vi "LinxServoGetChans.vi"(8 "Error In":errorcluster, 11 "LINX Resource":T1) -> (0 "Error Out":errorcluster, 1 "Num Servo Chans":i32, 2 "Servo Channels":u8[](array[numeric]), 3 "LINX Resource":T1)   [LabVIEW 2020, in "LMH-LINX.lvlib" / "Local IO.lvlib"]
uses:
  Local IO.lvlib
  Type Defs/LINX Ref.ctl
  Type Defs/Platform.ctl
  Device/Type Defs/LINX Device Config.ctl
  Type Defs/Interface.ctl
  Device/Type Defs/TCP Config.ctl
  Device/Type Defs/Channels.ctl
  Type Defs/Error Type.ctl
  LMH-LINX.lvlib
  <vilib>/MakerHub/LINX/Resources/liblinxdevice.dll
  Device/Device.lvlib
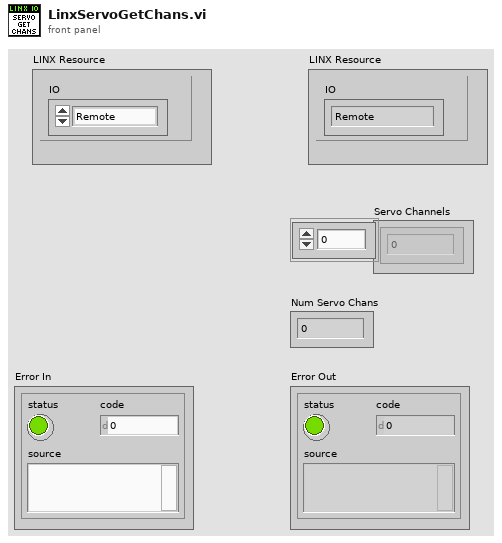
[diagram p1: front panel]
types:
  T1 = typedef "LMH-LINX.lvlib/LINX Ref.ctl" = cluster{"IO":T2, "LINX Device Config":T3}
  T2 = typedef "LMH-LINX.lvlib/Platform.ctl" = enum16{"Remote", "Local"}
  T3 = typedef "Device.lvlib/LINX Device Config.ctl" = cluster{"Interface":T4, "COM Port":refnum<visa-resource-name>, "TCP Configuration":T5, "Device Family":u8, "Device ID":u8, "Device Name":string, "TCP Ref":refnum<k5>, "Channels":T6}
  T4 = typedef "LMH-LINX.lvlib/Interface.ctl" = enum16{"Serial", "TCP"}
  T5 = typedef "Device.lvlib/TCP Config.ctl" = cluster{"IP Address":string, "Port":u16}
  T6 = typedef "LMH-LINX.lvlib/Channels.ctl" = cluster{"DI":u8[], "DO":u8[], "AI":u8[], "AO":u8[], "PWM":u8[], "QE":u8[], "UART":u8[], "I2C 2":u8[], "SPI":u8[], "CAN":u8[], "Servo":u8[], "AI Ref (V)":dbl, "AI Resolution (Bits)":u8, "AO Ref (V)":dbl, "AO Resolution (Bits)":u8}
  T7 = typedef "LMH-LINX.lvlib/Error Type.ctl" = enum16{"Unknown", "Timeout", "Corrupt Return Packet", "Unable To Connect", "Command Not Supported", "Channel DNE", "Invalid COM Config", "Firmware Version Mismatch", "myRIO Support", "CMD Specific Error", "Local IO Not Supported"}
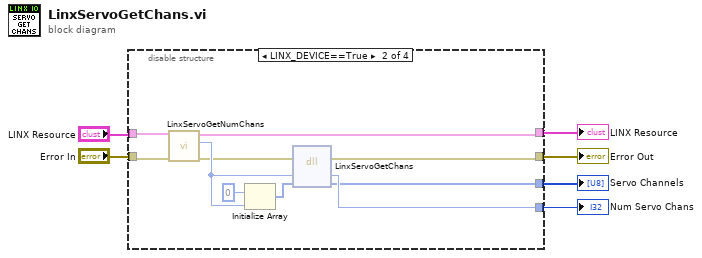
[diagram p0: block diagram]
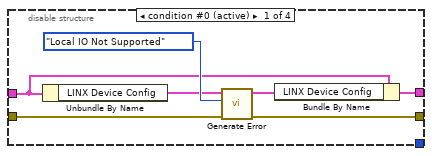
[diagram p2: hidden frame]
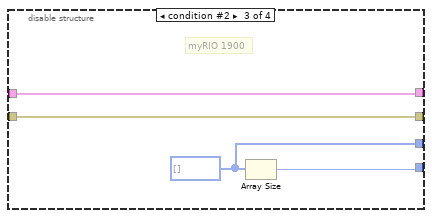
[diagram p3: hidden frame]
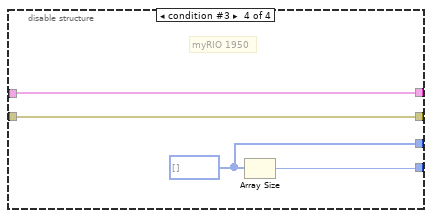
[diagram p4: hidden frame]
diagram:
  n1 = disable-structure shown="LINX_DEVICE==True" {
    disable-tunnel: [w7 w16 w26 w28] -> w3
    disable-tunnel: "LINX Resource" -> [w9 w19 w26 w28]
    disable-tunnel: "Error In" -> [w12 w18 w27 w31]
    disable-tunnel: [w11 w17 w27 w31] -> w5
    disable-tunnel: [_ w15 w25 w30] -> w2
    disable-tunnel: [_ w14 w24 w29] -> w1
    frame condition #0 (active) {
      n2 = Unbundle By Name(w9) -> ("LINX Device Config"=w10:T3)
      n3 = call "Generate Error.vi"("Error In"=w12, "Error Type"=Error_Type."Local IO Not Supported", "LINX Device Config"=w10) -> ("Error Out"=w11:errorcluster, "Dup LINX Device Config"=w8:T3)  [unwired: 7 in]
      n4 = Bundle By Name(cluster=w9, "LINX Device Config"=w8) -> (w7:T1)
    }
    frame condition #1 {
      n5 = call "LinxServoGetNumChans.vi"("Error In"=w18, "LINX Resource"=w19) -> ("Error Out"=w20:errorcluster, "ServoNumChans"=w22:u8, "LINX Resource"=w16:T1)  [unwired: 7 in]
      n6 = Initialize Array(u8 0 ("element"), w22) -> (w23:u8[])
      n7 = dll-call lib="E:/lv2019/dist/vi.lib/MakerHub/LINX/Resources/liblinxdevice.*" fn="LinxServoGetChans"(error in=w20, "numChans"=w22, "channels"=w23) -> (error out=w17:errorcluster, "numChans"=w15:u8, "channels"=w14:u8[])  [unwired: 3 in, 1 out]
    }
    frame condition #2 {
      w24 = u8[] [] ("Channels.I2C 2")
      # "myRIO 1900"
      n8 = Array Size(array=w24) -> (size(s)=w25:i32)
    }
    frame condition #3 {
      w29 = u8[] [] ("Channels.I2C 2")
      # "myRIO 1950"
      n9 = Array Size(array=w29) -> (size(s)=w30:i32)
    }
  }
  "LINX Resource" <- w3
  "Num Servo Chans" <- w2
  "Servo Channels" <- w1
  "Error Out" <- w5
